vi "SET_HEADING_ONEWHEEL.vi"(10 "argv":string[](array[string]), 11 "args":u8) -> ()   [LabVIEW 2015]
uses:
  Team Code/Robot Global Data.vi
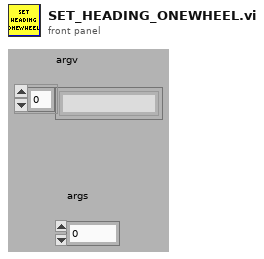
[diagram p1: front panel]
types:
  T1 = cluster{"Yaw":dbl, "Roll":dbl, "Pitch":dbl, "Heading":dbl, "Fused Heading":dbl}
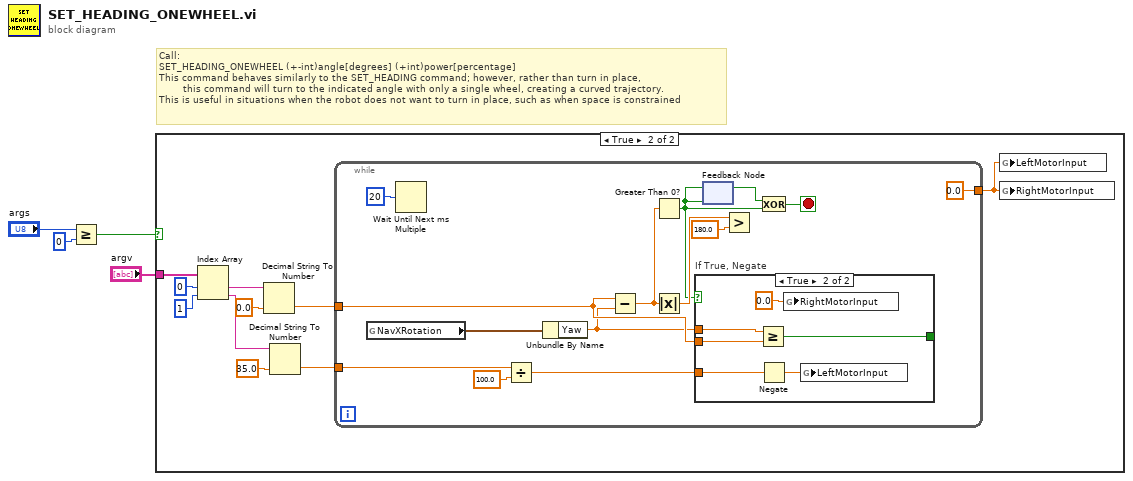
[diagram p0: block diagram]
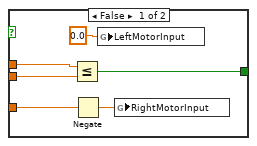
[diagram p3: hidden frame]
diagram:
  # "Call:\nSET_HEADING_ONEWHEEL (+-int)angle[degrees] (+int)power[percentage]\nThis command behaves similarly to the SET_HEADING command; however, rather than turn in place,\n        this command will turn to the indicated angle with only a single wheel, creating a curved trajectory.\nThis is useful in situations when the robot does not want to turn in place, such as when space is constrained"
  n1 = Greater Or Equal?(x="args", y=u8 0) -> (x >= y?=w1:bool)
  n2 = case shown="True" w1 {
    tunnel: "argv" -> [_ w7]
    frame False {
    }
    frame True {
      n3 = Index Array(array=w7, index #1=0 ("index"), index #2=1 ("index")) -> (element #1=w8:string, element #2=w6:string)
      n4 = Decimal String To Number(string=w8, default (0L)=0.0 ("default (0 I32)")) -> (number=w9:dbl)  [unwired: 2 out]
      n5 = Decimal String To Number(string=w6, default (0L)=35.0 ("default (0 I32)")) -> (number=w5:dbl)  [unwired: 2 out]
      n6 = while {
        tunnel: w9 -> [w20]
        tunnel: [0.0 ("LeftMotorInput")] -> w14
        tunnel: w5 -> [w25]
        stop <- w18 stop-if-true
        n7 = global read "Robot Global Data.vi" "NavXRotation"() -> (w16:T1)
        n8 = Wait Until Next ms Multiple(millisecond multiple=u32 20) -> ()  [unwired: 1 out]
        n9 = Divide(x=w25, y=100.0) -> (x/y=w21:dbl)
        n10 = Unbundle By Name(w16) -> ("Yaw"=w15:dbl)
        n11 = Subtract(x=w20, y=w15) -> (x-y=w24:dbl)
        n12 = Greater Than 0?(x=w24) -> (x > 0?=w17:bool)
        n13 = Absolute Value(x=w24) -> (abs(x)=w23:dbl)
        n14 = case "If True, Negate" shown="True" w17 {
          tunnel: w15 -> [w31 w37]
          tunnel: [w32 w38] -> _
          tunnel: w20 -> [w30 w36]
          tunnel: w21 -> [w34 w40]
          frame False {
            n15 = Less Or Equal?(x=w31, y=w30) -> (x <= y?=w32:bool)
            n16 = Negate(x=w34) -> (-x=w29:dbl)
            n17 = global write "Robot Global Data.vi" "LeftMotorInput"(0.0 ("LeftMotorInput")) -> ()
            n18 = global write "Robot Global Data.vi" "RightMotorInput"(w29) -> ()
          }
          frame True {
            n19 = Greater Or Equal?(x=w37, y=w36) -> (x >= y?=w38:bool)
            n20 = Negate(x=w40) -> (-x=w35:dbl)
            n21 = global write "Robot Global Data.vi" "RightMotorInput"(0.0 ("RightMotorInput")) -> ()
            n22 = global write "Robot Global Data.vi" "LeftMotorInput"(w35) -> ()
          }
        }
        n23 = feedback #1(w17) -> (w19:bool)
        n24 = feedback-in #1(w17) -> ()
        n25 = Greater?(x=w23, y=180.0) -> ()  [unwired: 1 out]
        n26 = Exclusive Or(1:w17, 2:w19) -> (0:w18:bool)
      }
      n27 = global write "Robot Global Data.vi" "LeftMotorInput"(w14) -> ()
      n28 = global write "Robot Global Data.vi" "RightMotorInput"(w14) -> ()
    }
  }
